vi "SteeringValidate.vi"() -> ()   [LabVIEW 2016]
uses:
  <vilib>/Platform/TimedLoop/XDataNode/timing_clust.ctl
  <vilib>/Platform/TimedLoop/XDataNode/nitl_modes.ctl
  <vilib>/Platform/TimedLoop/XDataNode/wakeup.ctl
  <vilib>/FPGAPlugInAG/roboRIO/niLvFpga_Open_roboRIO.vi
  <vilib>/rvi/interface/common/dynamic/niFpgaDynamicAddResources.vi
  <vilib>/FPGAPlugInAG/Dynamic/niLvFpga_Reset_Dynamic.vi
  <vilib>/FPGAPlugInAG/Dynamic/niLvFpga_Run_Dynamic.vi
  <vilib>/Utility/error.llb/Error Cluster From Error Code.vi
  <vilib>/rvi/errors/niLvFpgaAdjustHostInterfaceError.vi
  <vilib>/FPGAPlugInAG/Dynamic/niLvFpga_Abort_Dynamic.vi
  <vilib>/FPGAPlugInAG/Dynamic/niLvFpga_Close_Dynamic.vi
  <vilib>/rvi/interface/nirviOpenFPGA/nirviOpenFPGA.xnode
  FPGA Bitfiles/AutoBikeProject_FPGATarget_FPGASteeringVali_0ktHJXMggMw.lvbitx
  <vilib>/rvi/interface/nirviMethod/nirviMethod.xnode
  <vilib>/Platform/TimedLoop/XDataNode/XDataNode.xnode
  <vilib>/rvi/interface/nirviReadWriteControl/nirviReadWriteControl.xnode
  <vilib>/rvi/interface/nirviCloseFPGA/nirviCloseFPGA.xnode
  <vilib>/Platform/TimedLoop/XDataNode/XDNodeRunTimeDep.lvlib
  <vilib>/rvi/interface/Simulation/niFpgaSimulationCallBeginRW.vi
  NiFpgaLv.dll
panel:
  in  "Frequency of duty cycle 2":u32=40000
  out "duty cycle":dbl
  in  "pulse time (s)":dbl
  in  "Reset steering angle":bool
  out "Finished Late? [i-1]":bool
  in  "Stop":bool
  in  "Frequency of duty cycle":u32=40000
  in  "Direction":bool
  out "error out":errorcluster
  in  "error in (no error)":errorcluster
  # "Newton"
  # "Pulstid"
  # "DC"
  # "0.0\n0.05\n0.1\n0.15\n0.2\n0.25\n0.3\n0.35\n0.4\n0.45\n0.5\n0.55\n0.6\n0.65\n0.7\n0.75\n0.8\n0.85\n0.9"
  # "Front Panel Controls"
  # "CC"
  # "CW"
  # "100 = 0.2s\n200 = 0.4s\n300 = 0.6s\n400 = 0.8s\n500 = 1.0s"
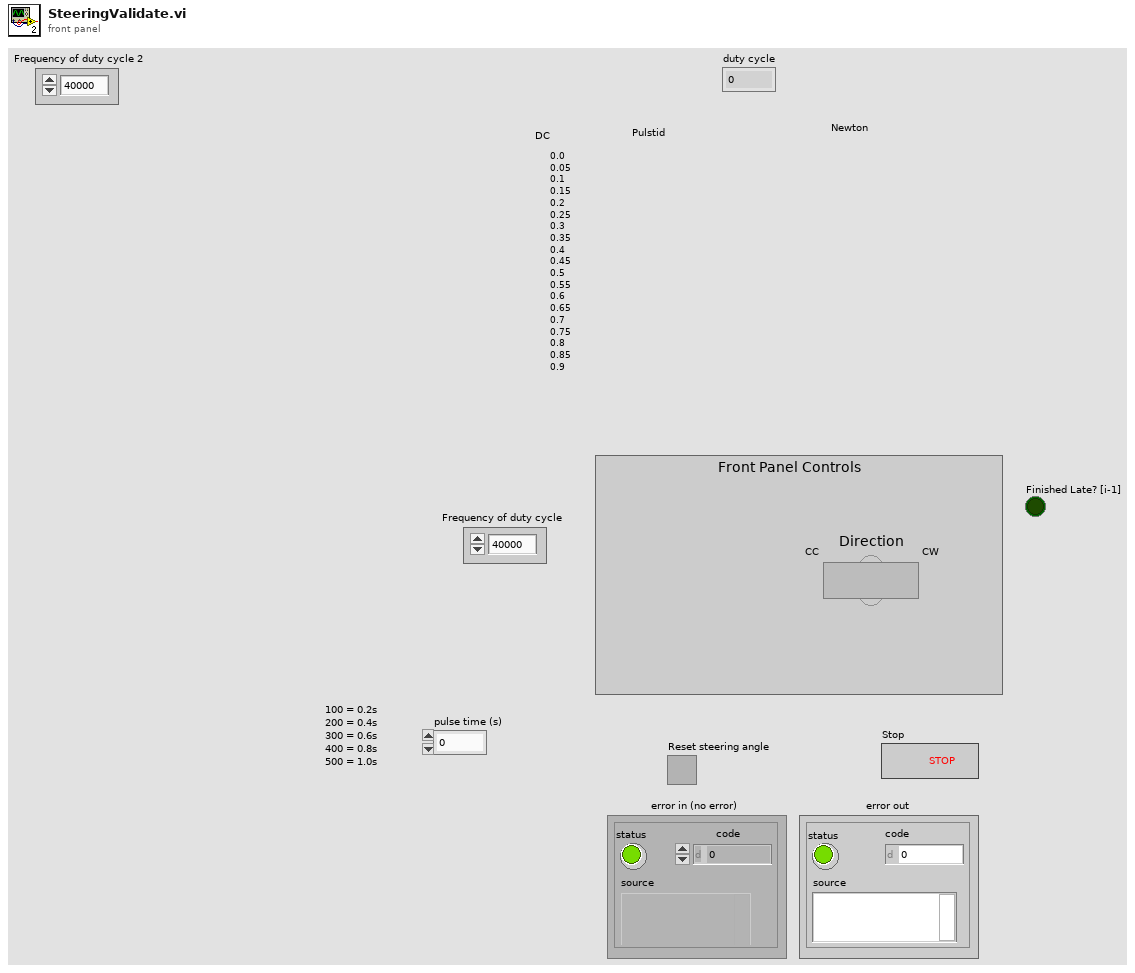
[diagram p1: front panel]
types:
  T1 = enum16{"open", "open or create", "create or replace", "create", "open (read-only)"}
  T2 = typedef "XDNodeRunTimeDep.lvlib/timing_clust.ctl" = cluster{"Expected End [f-1]":u64, "Actual End [f-1]":u64, "Finished Late? [f-1]":bool, "Expected End [i-1]":u64, "Actual End [i-1]":u64, "Finished Late? [i-1]":bool, "Expected Start [i]":u64, "Actual Start [i]":u64, "Expected Start [f]":u64, "Actual Start [f]":u64, "Source Name":string, "Structure Name":string, "Period":i64, "Deadline":i64, "Offset":i64, "Start":i64, "Priority":i32, "Timeout":i32, "Mode":T3, "Wakeup Reason":T4, "Error":errorcluster, "Source Type":string, "Secondary Source Type":string, "Global End Time":u64, "Global Start Time":u64, "Frame Duration":u64, "Iteration Duration":u64, "Assigned CPU":i32, "I/O Scan Engine Mode":u32}
  T3 = typedef "XDNodeRunTimeDep.lvlib/nitl_modes.ctl" = enum32{"No Change", "Process missed periods, maintain original phase", "Discard missed periods, maintain original phase", "Process missed periods, ignore original phase", "Discard missed periods, ignore original phase"}
  T4 = typedef "XDNodeRunTimeDep.lvlib/wakeup.ctl" = enum32{"Normal", "Aborted", "Asynchronous wakeup", "Timing source error", "Timed loop error", "Timeout"}
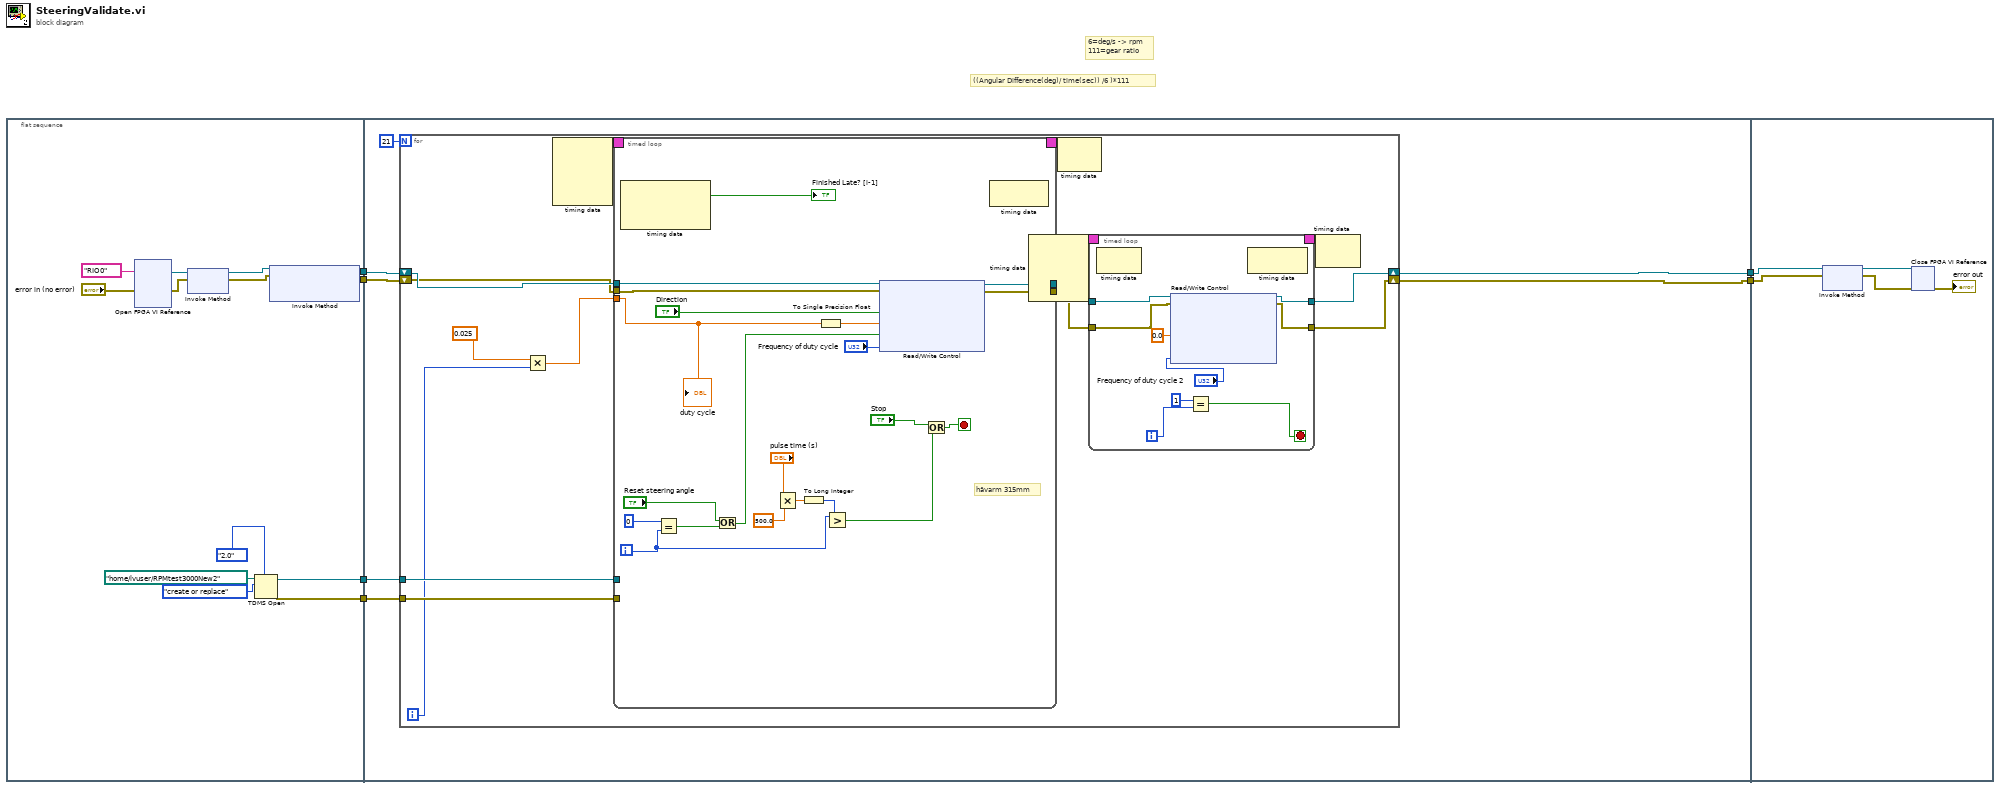
[diagram p0: block diagram]
diagram:
  # "6=deg/s -> rpm\n111=gear ratio"
  # "((Angular Difference(deg)/ time(sec)) /6 )*111"
  n1 = flat-sequence {
    tunnel: [w10] -> w6
    tunnel: [w9] -> w5
    tunnel: [w12] -> w4
    tunnel: [w11] -> w3
    tunnel: w6 -> [w23]
    tunnel: w5 -> [w22]
    tunnel: w4 -> [w25]
    tunnel: w3 -> [w24]
    tunnel: [w26] -> w2
    tunnel: [w21] -> w1
    tunnel: w2 -> [w82]
    tunnel: w1 -> [w81]
    frame #0 {
      n2 = xnode "Open FPGA VI Reference"("error in"="error in (no error)", "resource name"=tag "RIO0") -> ("FPGA VI Reference Out"=w17:refnum<k20>, "error out"=w16:errorcluster)
      n3 = xnode "Invoke Method"("FPGA VI Reference In"=w17, "error in"=w16) -> ("FPGA VI Reference Out"=w7:refnum<k20>, "error out"=w8:errorcluster)
      n4 = TDMS Open(7:enum16{"1.0", "2.0"}."2.0" ("file format version (2.0)"), 10:T1."create or replace" ("operation (0:open)"), 11:path "/home/lvuser/RPMtest3000New2" ("file path")) -> (0:w11:errorcluster, 3:w12:refnum<k34>)  [unwired: 4 in]
      n5 = xnode "Invoke Method"("FPGA VI Reference In"=w7, "error in"=w8) -> ("FPGA VI Reference Out"=w10:refnum<k20>, "error out"=w9:errorcluster)  [unwired: 1 in]
    }
    frame #1 {
      n6 = for {
        N: 21 -> [_]
        tunnel: w25 -> [w39]
        tunnel: w24 -> [w38]
        shift-right: [w29] -> w26
        shift-left: w23 -> [w37]
        shift-right: [w27] -> w21
        shift-left: w22 -> [w36]
        i -> [w35]
        n7 = Multiply(x=0.025, y=w35) -> (x*y=w33:dbl)
        n8 = node-c288() -> (w41:T2)  [unwired: 4 in]
        n9 = timed-loop {
          timing: w41 -> [_]
          timing-out: [_] -> w40
          tunnel: [w69] -> w30
          tunnel: [w68] -> w28
          tunnel: w37 -> [w75]
          tunnel: w36 -> [w74]
          tunnel: w39 -> [_]
          tunnel: w38 -> [_]
          tunnel: w33 -> [w55]
          i -> [w63]
          stop <- w62 stop-if-true
          # "hävarm 315mm"
          n10 = node-c288() -> (→"Finished Late? [i-1]":bool)  [unwired: 1 in, 2 out]
          n11 = Equal?(x=0, y=w63) -> (x = y?=w66:bool)
          n12 = Or(x="Reset steering angle", y=w66) -> (x .or. y?=w65:bool)
          n13 = Multiply(x="pulse time (s)", y=500.0) -> (x*y=w58:dbl)
          n14 = To Long Integer(number=w58) -> (32bit integer=w59:i32)
          n15 = To Single Precision Float(number=w55) -> (single precision float=w71:sgl)
          n16 = Greater?(x=w63, y=w59) -> (0:w60:bool)
          n17 = xnode "Read/Write Control"("FPGA VI Reference In"=w75, "error in"=w74, "Direction"="Direction", "Front Panel Duty Cycle"=w71, "Reset counter"=w65, "Freq"="Frequency of duty cycle") -> ("FPGA VI Reference Out"=w69:refnum<k20>, "error out"=w68:errorcluster)  [unwired: 1 out]
          n18 = Or(x="Stop", y=w60) -> (x .or. y?=w62:bool)
          n19 = node-c288() -> ()  [unwired: 1 in, 1 out]
          "duty cycle" <- w55
        }
        n20 = node-c288() -> (w32:T2)  [unwired: 4 in]
        n21 = node-c288(w40) -> ()  [unwired: 1 out]
        n22 = timed-loop {
          timing: w32 -> [_]
          timing-out: [_] -> w31
          tunnel: w30 -> [w50]
          tunnel: [w48] -> w29
          tunnel: w28 -> [w49]
          tunnel: [w47] -> w27
          i -> [w45]
          stop <- w44 stop-if-true
          n23 = node-c288() -> ()  [unwired: 1 in, 1 out]
          n24 = xnode "Read/Write Control"("FPGA VI Reference In"=w50, "error in"=w49, "Front Panel Duty Cycle"=sgl 0.0, "Freq"="Frequency of duty cycle 2") -> ("FPGA VI Reference Out"=w48:refnum<k20>, "error out"=w47:errorcluster)  [unwired: 2 in, 1 out]
          n25 = Equal?(x=1, y=w45) -> (x = y?=w44:bool)
          n26 = node-c288() -> ()  [unwired: 1 in, 1 out]
        }
        n27 = node-c288(w31) -> ()  [unwired: 1 out]
      }
    }
    frame #2 {
      n28 = xnode "Invoke Method"("FPGA VI Reference In"=w82, "error in"=w81) -> ("FPGA VI Reference Out"=w84:refnum<k20>, "error out"=w85:errorcluster)
      n29 = xnode "Close FPGA VI Reference"("FPGA VI Reference In"=w84, "error in"=w85) -> ("error out"=→"error out":errorcluster)
    }
  }
